vi "Stop Core.vi"(10 "final error code":i32, 11 "Signal Generation in":refnum<class "Signal Generation.lvclass">) -> (3 "Signal Generation out":refnum<class "Signal Generation.lvclass">)   [LabVIEW 2020, in "Signal Generation.lvlib" / "Signal Generation.lvclass"]
doc: "(<B>Filename</B>: Actor Framework.lvlib:Actor.lvclass:Stop Core.vi)\n\nDefines what the actor does before it stops. Use the <B>final error code</B> input to determine whether the actor shut down in response to an error.\n\nBy default, this method passes the Stop message along to all auto-stop nested actors. A descendant class may override this method to define additional behavior, such as shutting down any processes the actor initiated in its override of the Actor Core method."
uses:
  Signal Generation.lvclass
  Signal Generation.lvclass/Signal Generation.ctl
  <vilib>/ActorFramework/Actor/Actor.lvclass
  Signal Generation.lvlib
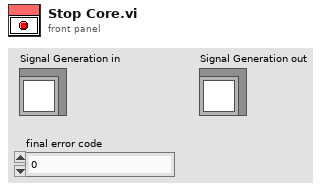
[diagram p1: front panel]
types:
  T1 = cluster{"Start/Stop":refnum<user-event>, "Exit":refnum<user-event>, "Signal Parameters":refnum<user-event>}
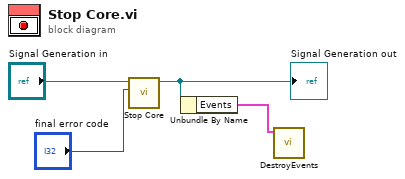
[diagram p0: block diagram]
diagram:
  n1 = call-parent "Stop Core.vi"("final error code"="final error code", "Actor in"="Signal Generation in") -> ("Actor out"=w2:refnum<class "Signal Generation.lvclass">)  [unwired: 9 in]
  "Signal Generation out" <- w2
  n2 = Unbundle By Name(w2) -> ("Events"=w1:T1)
  n3 = call "DestroyEvents.vi"("Events"=w1) -> ()  [unwired: 10 in, 1 out]
